vi "Launch DAQ Interface.vi"(8 "error in (no error)":errorcluster, 11 "Guardian in":refnum<class "Guardian.lvclass">) -> (0 "error out":errorcluster, 3 "Guardian out":refnum<class "Guardian.lvclass">)   [LabVIEW 2026, in "TALOS.lvlib" / "Guardian.lvlib" / "Guardian.lvclass"]
uses:
  Guardian.lvclass
  C:/LabVIEW Code/TALOS/talos/Ancestor/Ancestor/Ancestor.lvclass
  C:/LabVIEW Code/TALOS/builds/Actor Framework PPL/Actor Framework.lvlibp/1abvi3w/vi.lib/ActorFramework/Actor/Actor.lvclass
  Ancestor/Ancestor/Ancestor.lvclass/Ancestor.ctl
  Guardian Messages/Launch uService Msg/Launch uService Msg.lvclass/Launch uService Msg.ctl
  Ancestor/Ancestor/Read ID.vi
  Support VIs/Generate Error.vi
  FGV/Error Memory/Get Error Description.vi
  Support VIs/Get PC name.vi
  Support VIs/Get Class Name.vi
  <vilib>/Utility/error.llb/Clear Errors.vi
  FGV/Error Memory/Error Memory Core.vi
  <vilib>/AdvancedString/Delimited String to 1D String Array.vi
  <vilib>/AdvancedString/Delimited String to 1D String Array (string).vi
  Support VIs/Circus Root Path.vi
  FGV/Error Memory/Error Crt Lvl checker.vi
  FGV/Error Memory/Error Memory Core.vi/40c8088d-b597-4017-91af-faa98e00292e.vi
  FGV/Error Memory/Error Memory Core.vi/d4a3ab98-063c-4e44-b43d-fbdcfe6c2be2.vi
  Support VIs/Global Memory.vi
  <vilib>/Utility/LVClass/Get LV Class Name.vi
  Support VIs/Is in Packed Library.vi
  Support VIs/TALOS Root path.vi
  Support VIs/Read CSV worksheet.vi
  Support VIs/Global Constants.vi
  <vilib>/Utility/error.llb/General Error Handler.vi
  <vilib>/Utility/config.llb/Open Config Data.vi
  <vilib>/Utility/config.llb/Get Section Names.vi
  <vilib>/Utility/config.llb/Get Key Names.vi
  <vilib>/Utility/config.llb/Read Key.vi
  <vilib>/Utility/config.llb/Read Key (String).vi
  <vilib>/Utility/config.llb/Close Config Data.vi
  builds/Actor Framework PPL/Actor Framework.lvlibp/1abvi3w/vi.lib/ActorFramework/Message Enqueuer/Enqueue.vi
  Ancestor/Ancestor/Ancestor.lvclass
  <vilib>/Comparison/Equal/Equal Functor/Equal Functor.lvclass
  Guardian Messages/Launch uService Msg/Launch uService Msg.lvclass
  builds/Actor Framework PPL/Actor Framework.lvlibp/1abvi3w/vi.lib/ActorFramework/Actor/Actor.lvclass
  TALOS.lvlib
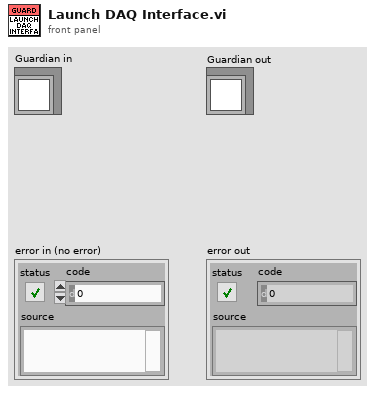
[diagram p1: front panel]
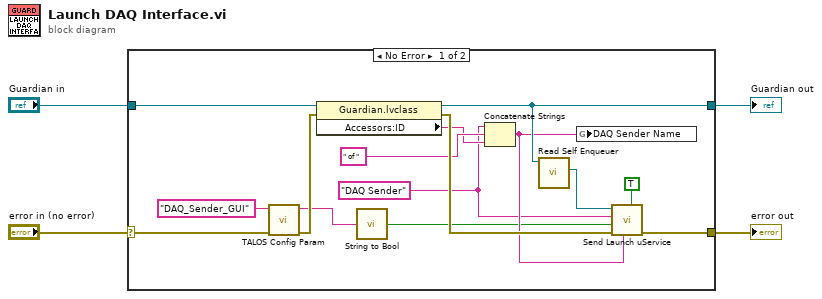
[diagram p0: block diagram]
diagram:
  n1 = case shown="No Error" "error in (no error)" {
    selector: "error in (no error)" -> [w9 w21]
    tunnel: "Guardian in" -> [w16 w20]
    tunnel: [w18 w21] -> w2
    tunnel: [w14 w20] -> w1
    frame No Error {
      w10 = "DAQ Sender"
      n2 = call "TALOS Config Param.vi"("error in (no error)"=w9, "Parameter Name"="DAQ_Sender_GUI") -> ("error out"=w8:errorcluster, "Output"=w6:string)  [unwired: 8 in]
      n3 = property class="Guardian.lvclass"(reference=w16, error in=w8) -> (reference out=w14:refnum<class "Guardian.lvclass">, error out=w15:errorcluster, "Accessors:ID"=w12:string)
      n4 = call "String to Bool.vi"("String"=w6) -> ("Boolean"=w5:bool)
      n5 = Concatenate Strings(w10, " of ", w12) -> (w11:string)
      n6 = call "Read Self Enqueuer.vi"("Actor"=w14) -> ("Self Enqueuer"=w19:refnum<class "Message Enqueuer.lvclass">)  [unwired: 10 in]
      n7 = global write "Global Memory.vi" "DAQ Sender Name"(w11) -> ()
      n8 = call "Send Launch uService.vi"("Highlander?"=TRUE, "uService ID"=w11, "error in (no error)"=w15, "GUI?"=w5, "uService Class Name"=w10, "Message Enqueuer"=w19) -> ("error out"=w18:errorcluster)  [unwired: 4 in, 1 out]
    }
    frame Error {
    }
  }
  "error out" <- w2
  "Guardian out" <- w1
